vi "OpenCVCam_GetPicture.vi"(8 "ErrorIn":errorcluster, 10 "CmdData":variant, 11 "OpenCVCamIn":refnum<class>) -> (0 "ErrorOut":errorcluster, 2 "ReplyData":variant, 3 "OpenCVCamOut":refnum<class>, 4 "Exit":bool)   [LabVIEW 2021, in "OpenCVCam.lvclass"]
uses:
  OpenCVCam.lvclass
  OpenCVCam_UiCallBackEvents.ctl
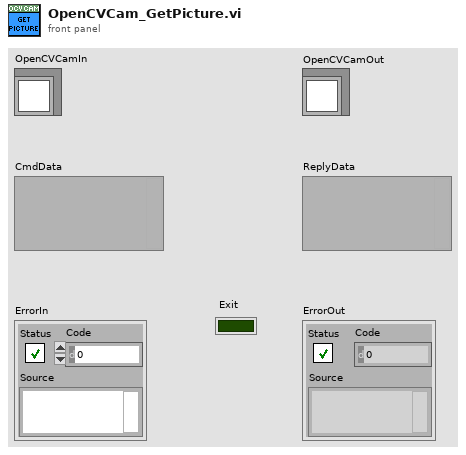
[diagram p1: front panel]
types:
  T1 = typedef "OpenCVCam.lvclass/OpenCVCam_UiCallBackEvents.ctl" = enum16{"Default", "PersistentDataUpdated", "NewPicture", "Worker 1: Do Something"}
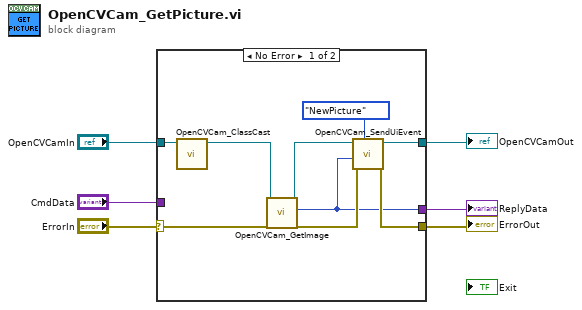
[diagram p0: block diagram]
diagram:
  n1 = case shown="No Error" "ErrorIn" {
    selector: "ErrorIn" -> [w15 w18]
    tunnel: [w14 w18] -> w5
    tunnel: [w9 w17] -> w3
    tunnel: "CmdData" -> [_ w17]
    tunnel: "OpenCVCamIn" -> [w12 w16]
    tunnel: [w10 w16] -> w1
    frame No Error {
      n2 = call "OpenCVCam_ClassCast.vi"("OpenCVCamIn"=w12) -> ("OpenCVCamOut"=w11:refnum<class "OpenCVCam.lvclass">)  [unwired: 10 in]
      n3 = call "OpenCVCam_GetImage.vi"("ErrorIn"=w15, "OpenCVCamIn"=w11) -> ("ErrorOut"=w13:errorcluster, "NewPicture"=w9:picture, "OpenCVCamOut"=w7:refnum<class "OpenCVCam.lvclass">)  [unwired: 7 in]
      n4 = call "OpenCVCam_SendUiEvent.vi"("UiEventNames"=OpenCVCam_UiCallBackEvents."NewPicture", "ErrorIn"=w13, "Data"=w9, "OpenCVCamIn"=w7) -> ("ErrorOut"=w14:errorcluster, "OpenCVCamOut"=w10:refnum<class "OpenCVCam.lvclass">)  [unwired: 6 in]
    }
    frame Error {
    }
  }
  "ErrorOut" <- w5
  "OpenCVCamOut" <- w1
  "ReplyData" <- w3
